vi "Refresh.vi"(8 "error in (no error)":errorcluster, 10 "Debug Log":T1[](array[typedef]), 11 "Chronological List In":refnum<class "Chronological List.lvclass">) -> (0 "error out":errorcluster, 3 "Chronological List Out":refnum<class "Chronological List.lvclass">)   [LabVIEW 2020, in "Chronological List.lvclass"]
uses:
  Chronological List.lvclass
  Debugger/TypeDefs/Debug Data.ctl
  Chronological List.lvclass/Chronological List.ctl
  Debugger/Debugger.lvclass
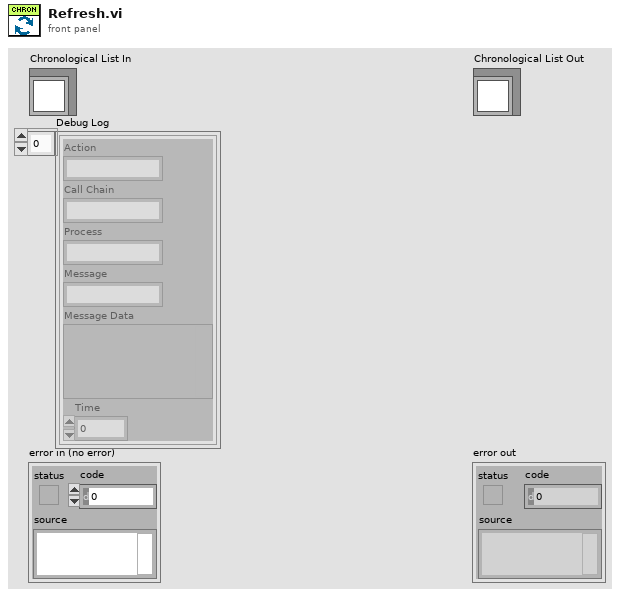
[diagram p1: front panel]
types:
  T1 = typedef "Debugger.lvclass/Debug Data.ctl" = cluster{"Action":string, "Call Chain":string, "Process":string, "Message":string, "Message Data":variant, "Time":u32}
  T2 = typedef "LVRowAndColumnUnsignedTypeDef.ctl" = cluster{"Row":u32, "Column":u32}
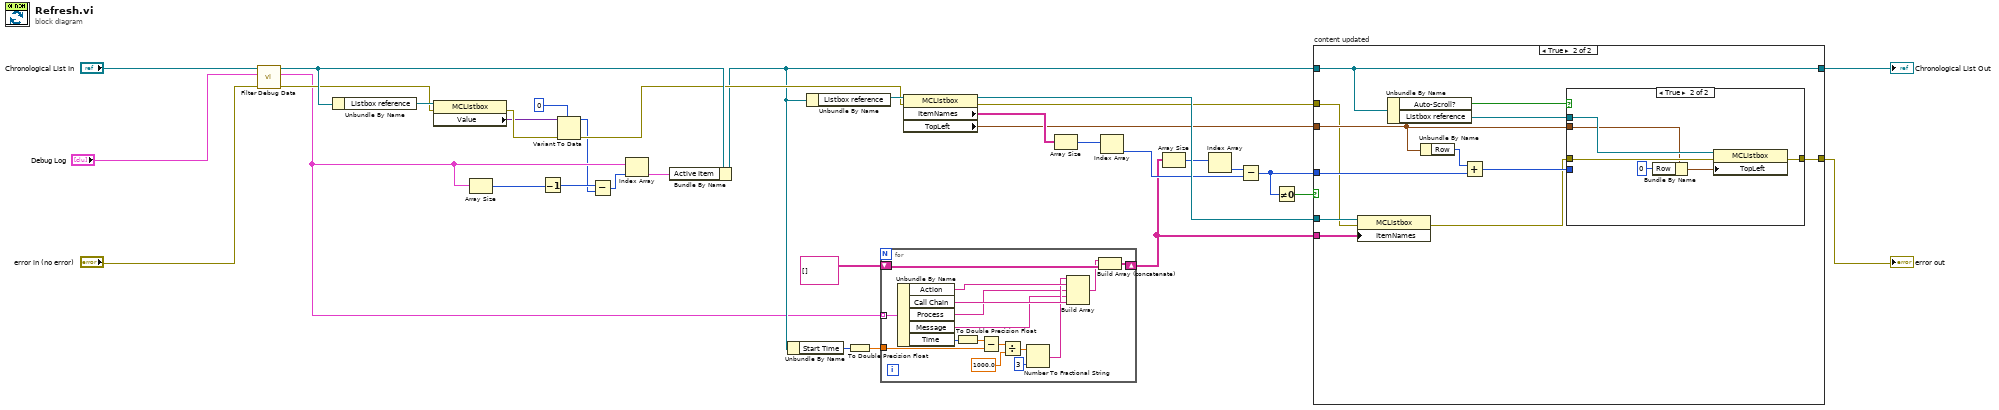
[diagram p0: block diagram]
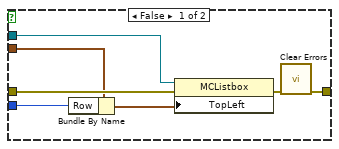
[diagram p3: hidden frame]
diagram:
  n1 = call "Filter Debug Data.vi"("error in (no error)"="error in (no error)", "Debug Log"="Debug Log", "Chronological List In"="Chronological List In") -> ("error out"=w15:errorcluster, "Filtered Debug Log"=w9:T1[], "Chronological List Out"=w19:refnum<class "Chronological List.lvclass">)  [unwired: 6 in]
  n2 = Unbundle By Name(w19) -> ("Listbox reference"=w18:refnum<vi>)
  n3 = property on="Property Node" class="MCListbox"(reference=w18, error in=w15) -> (error out=w17:errorcluster, "Value"=w16:variant)  [unwired: 1 out]
  n4 = Array Size(array=w9) -> (size(s)=w8:i32)
  n5 = Decrement(x=w8) -> (x-1=w7:i32)
  n6 = Variant To Data(error in=w17, type=0, Variant=w16) -> (data=w6:i32, error out=w14:errorcluster)
  n7 = Subtract(x=w7, y=w6) -> (x-y=w5:i32)
  n8 = Index Array(array=w9, index=w5) -> (element=w12:T1)
  n9 = Bundle By Name(cluster=w19, "Active Item"=w12) -> (w13:refnum<class "Chronological List.lvclass">)
  n10 = Unbundle By Name(w13) -> ("Start Time"=w22:i32)
  n11 = Unbundle By Name(w13) -> ("Listbox reference"=w25:refnum<vi>)
  n12 = To Double Precision Float(number=w22) -> (double precision float=w21:dbl)
  n13 = for {
    tunnel: w9 -> [w39] mode=indexing
    tunnel: w21 -> [w38]
    shift-right: [w36] -> w10
    shift-left: string[][] [] -> [w37]
    n14 = Unbundle By Name(w39) -> ("Action"=w49:string, "Call Chain"=w50:string, "Process"=w41:string, "Message"=w40:string, "Time"=w48:u32)
    n15 = To Double Precision Float(number=w48) -> (double precision float=w42:dbl)
    n16 = Subtract(x=w42, y=w38) -> (x-y=w47:dbl)
    n17 = Divide(x=w47, y=1000.0) -> (x/y=w45:dbl)
    n18 = Number To Fractional String(number=w45, precision (6)=i16 3) -> (F-format string=w43:string)  [unwired: 2 in]
    n19 = Build Array(w43, w49, w41, w40, w50) -> (w35:string[])
    n20 = Build Array (concatenate)(w35, w37) -> (w36:string[][])
  }
  n21 = property on="Property Node" class="MCListbox"(reference=w25, error in=w14) -> (reference out=w34:refnum<vi>, error out=w4:errorcluster, "ItemNames"=w33:string[][], "TopLeft"=w28:T2)
  n22 = Array Size(array=w33) -> (size(s)=w31:i32[])
  n23 = Index Array(array=w31) -> (element=w30:i32)  [unwired: 1 in]
  n24 = Array Size(array=w10) -> (size(s)=w32:i32[])
  n25 = Index Array(array=w32) -> (element=w29:i32)  [unwired: 1 in]
  n26 = Subtract(x=w29, y=w30) -> (x-y=w2:i32)
  n27 = Not Equal To 0?(x=w2) -> (x != 0?=w1:bool)
  n28 = case "content updated" shown="True" w1 {
    tunnel: w34 -> [_ w63]
    tunnel: w28 -> [_ w60]
    tunnel: [w52 w58] -> w26
    tunnel: w13 -> [w51 w53]
    tunnel: w10 -> [_ w57]
    tunnel: w4 -> [w52 w55]
    tunnel: [w51 w53] -> w3
    tunnel: w2 -> [_ w56]
    frame False {
    }
    frame True {
      n29 = property on="Property Node" class="MCListbox"(reference=w63, error in=w55, "ItemNames"=w57) -> (error out=w59:errorcluster)  [unwired: 1 out]
      n30 = Unbundle By Name(w53) -> ("Auto-Scroll?"=w54:bool, "Listbox reference"=w64:refnum<vi>)
      n31 = Unbundle By Name(w60) -> ("Row"=w62:u32)
      n32 = Add(x=w62, y=w56) -> (x+y=w61:u32)
      n33 = case shown="True" w54 {
        tunnel: w64 -> [w71 w77]
        tunnel: w59 -> [w70 w76]
        tunnel: [w65 w75] -> w58
        tunnel: w61 -> [w68 _]
        tunnel: w60 -> [w67 w74]
        frame False {
          n34 = Bundle By Name(cluster=w67, "Row"=w68) -> (w66:T2)
          n35 = property on="Property Node" class="MCListbox"(reference=w71, error in=w70, "TopLeft"=w66) -> (error out=w69:errorcluster)  [unwired: 1 out]
          n36 = call <vilib>:"Clear Errors.vi"("error in (no error)"=w69) -> ("error out"=w65:errorcluster)  [unwired: 5 in, 1 out]
        }
        frame True {
          n37 = Bundle By Name(cluster=w74, "Row"=u32 0) -> (w72:T2)
          n38 = property on="Property Node" class="MCListbox"(reference=w77, error in=w76, "TopLeft"=w72) -> (error out=w75:errorcluster)  [unwired: 1 out]
        }
      }
    }
  }
  "error out" <- w26
  "Chronological List Out" <- w3
